vi "Pilot proved.vi"(8 "error in (no error)":errorcluster, 9 "Boiler Simulation Controls":T1 {"Flame Sensor Value (%)" min=0.0 max=100.0 scale=0.0..100.0}, 10 "Indicator states in":T3 {"Time Count" format="%.2g"}, 11 "Runtime statuses in":T2) -> (0 "error out":errorcluster, 2 "Indicator states out":T3 {"Time Count" format="%.2g"}, 3 "Runtime statuses out":T2)   [LabVIEW 2014]
doc: "Updates runtime statuses and Boiler indicator states after pilot is proved"
uses:
  Controls/Boiler Status Indicators.ctl
  Controls/Boiler runtime status indicators.ctl
  Controls/Boiler Simulation Controls.ctl
  Controls/Log file FGV action enum.ctl
  Controls/Log event enum.ctl
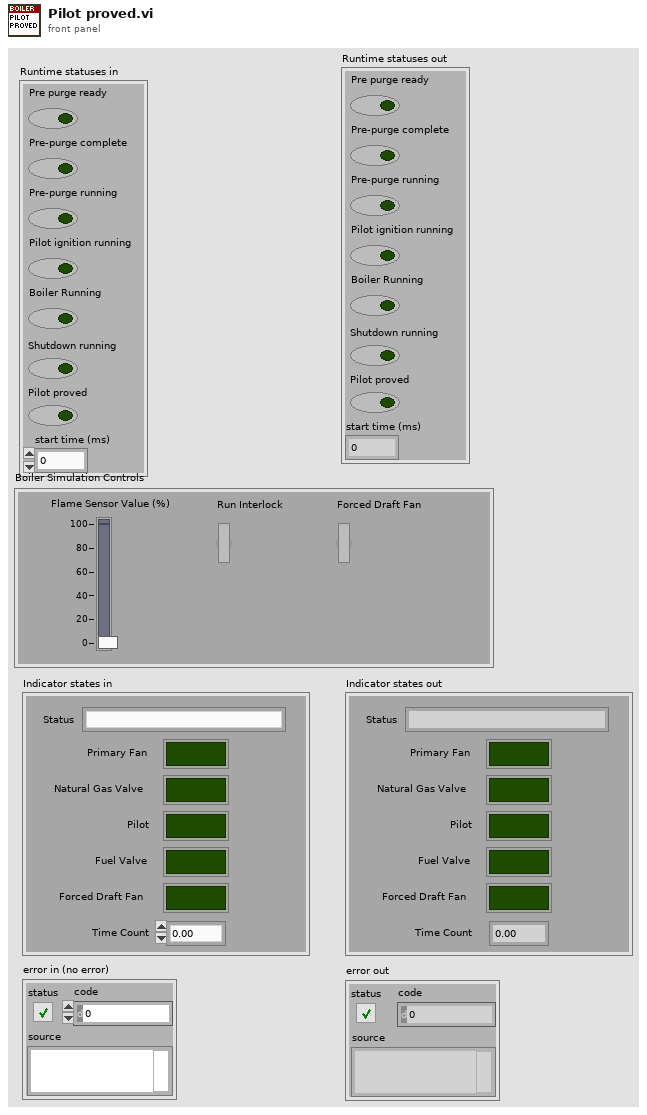
[diagram p1: front panel]
types:
  T1 = typedef "Boiler Simulation Controls.ctl" = cluster{"Flame Sensor Value (%)":dbl, "Run Interlock":bool, "Forced Draft Fan":bool}
  T2 = typedef "Boiler runtime status indicators.ctl" = cluster{"Pre purge ready":bool, "Pre-purge complete":bool, "Pre-purge running":bool, "Pilot ignition running":bool, "Boiler Running":bool, "Shutdown running":bool, "Pilot proved":bool, "start time (ms)":u32}
  T3 = typedef "Boiler Status Indicators.ctl" = cluster{"Status":string, "Primary Fan":bool, "Natural Gas Valve":bool, "Pilot":bool, "Fuel Valve":bool, "Forced Draft Fan":bool, "Time Count":dbl}
  T4 = typedef "Log event enum.ctl" = enum16{"Boiler Initialized", "Boiler Ready", "Start Pre-Purge", "Pre-Purge Complete", "Pilot ON", "Pilot proved", "Forced Draft Fan ON", "Boiler Running", "Start Shutdown Purge", "Shutdown Purge Complete"}
  T5 = typedef "Log file FGV action enum.ctl" = enum16{"open log file", "log event", "close log file"}
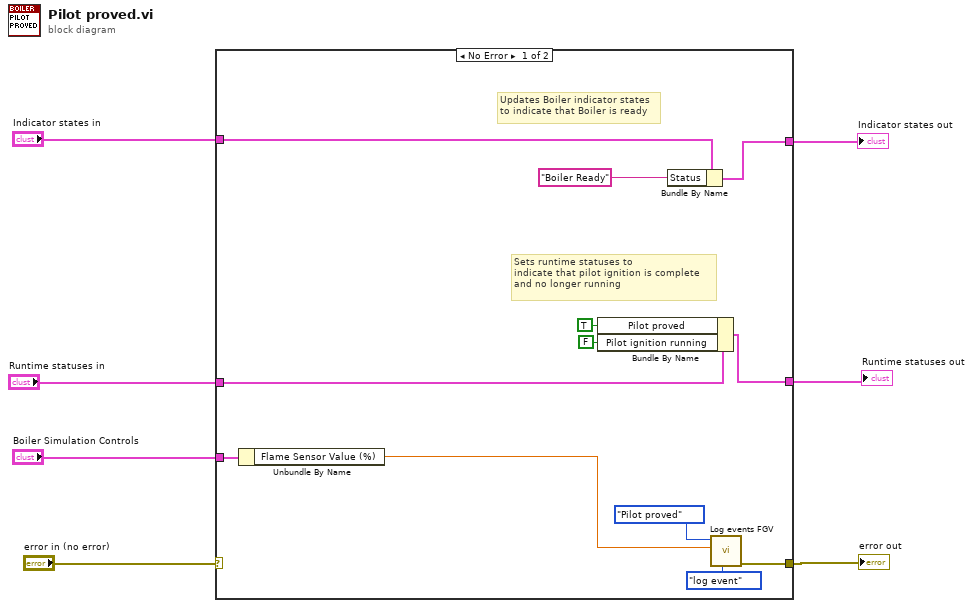
[diagram p0: block diagram]
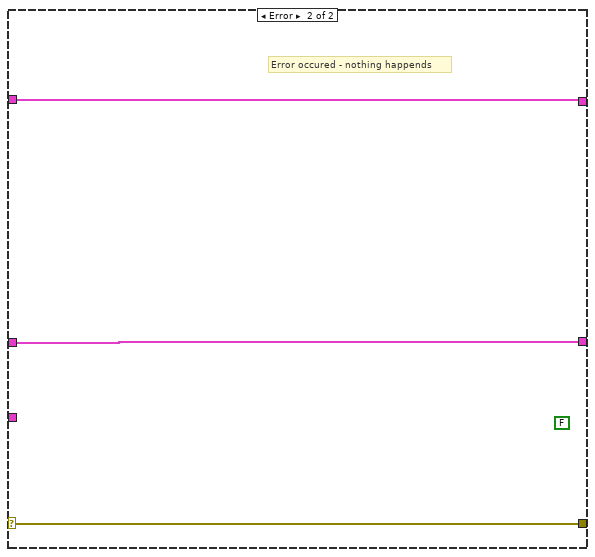
[diagram p2: hidden frame]
diagram:
  n1 = case shown="No Error" "error in (no error)" {
    selector: "error in (no error)" -> [_ w22]
    tunnel: [w10 w22] -> w6
    tunnel: "Runtime statuses in" -> [w17 w20]
    tunnel: "Indicator states in" -> [w19 w21]
    tunnel: [w18 w21] -> w3
    tunnel: [w16 w20] -> w2
    tunnel: "Boiler Simulation Controls" -> [w9 _]
    frame No Error {
      # "Sets runtime statuses to\nindicate that pilot ignition is complete\nand no longer running"
      # "Updates Boiler indicator states\nto indicate that Boiler is ready"
      n2 = Unbundle By Name(w9) -> ("Flame Sensor Value (%)"=w8:dbl)
      n3 = Bundle By Name(cluster=w17, "Pilot proved"=TRUE ("Pre-purge complete"), "Pilot ignition running"=FALSE ("Pre purge ready")) -> (w16:T2)
      n4 = Bundle By Name(cluster=w19, "Status"="Boiler Ready") -> (w18:T3)
      n5 = call "Log events FGV.vi"("action"=Log_file_FGV_action_enum."log event", "Event data"=w8, "Log event"=Log_event_enum."Pilot proved") -> ("error out"=w10:errorcluster)  [unwired: 8 in]
    }
    frame Error {
      (unwired) FALSE
      # "Error occured - nothing happends"
    }
  }
  "Indicator states out" <- w3
  "error out" <- w6
  "Runtime statuses out" <- w2
